vi "Create All Message Queues Sample Panel.vi"(8 "error in (no error)":cluster{"状态":bool, "代码":i32, "源":string} caption="错误输入（无错误）") -> (0 "error out":cluster{"状态":bool, "代码":i32, "源":string} caption="错误输出", 3 "消息队列":T1)   [LabVIEW 2015, in "Message Queue.lvlib"]
doc: "本VI用于创建应用程序所需的所有消息队列。如应用程序需要两个以上消息队列，可右键单击上面的“消息队列”常量并选择打开自定义类型，将新的消息队列添加至该自定义类型，然后通过本VI进行初始化。"
uses:
  Message Queue.lvlib
  All Message Queues Sample Panel.ctl
  Message Cluster.ctl
  Enqueue Message (Single).vi
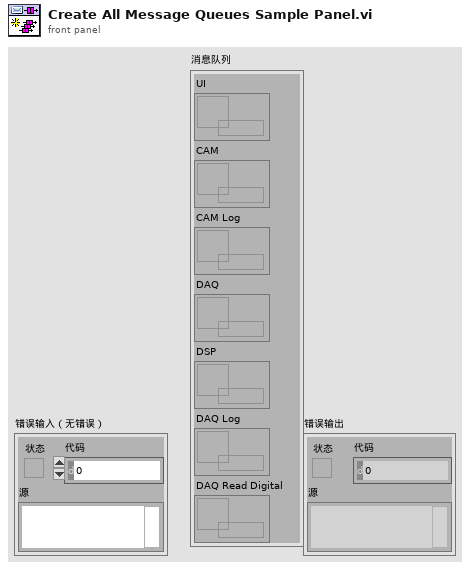
[diagram p1: front panel]
types:
  T1 = typedef "Message Queue.lvlib/All Message Queues Sample Panel.ctl" = cluster{"UI":refnum<queue>, "CAM":refnum<queue>, "CAM Log":refnum<queue>, "DAQ":refnum<queue>, "DSP":refnum<queue>, "DAQ Log":refnum<queue>, "DAQ Read Digital":refnum<queue>}
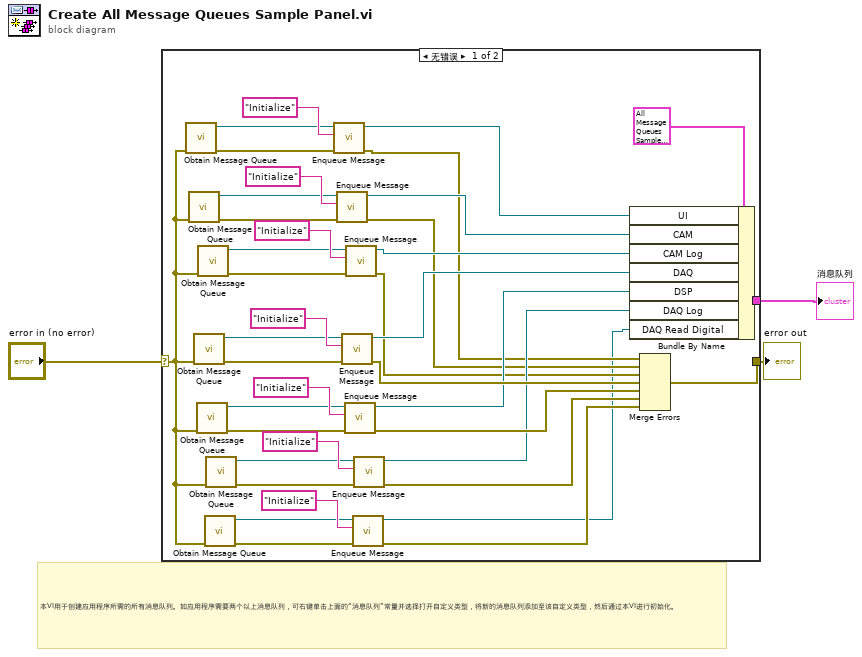
[diagram p0: block diagram]
diagram:
  # "本VI用于创建应用程序所需的所有消息队列。如应用程序需要两个以上消息队列，可右键单击上面的“消息队列”常量并选择打开自定义类型，将新的消息队列添加至该自定义类型，然后通过本VI进行初始化。"
  n1 = case shown="无错误" "error in (no error)" {
    selector: "error in (no error)" -> [w6 w43]
    tunnel: [w35 w43] -> w3
    tunnel: [w42 _] -> w1
    frame No Error {
      n2 = call "Obtain Message Queue.vi"("error in (no error)"=w6) -> ("error out"=w24:cluster{"状态":bool, "代码":i32, "源":string}, "消息队列"=w22:refnum<queue>)  [unwired: 9 in]
      n3 = call "Obtain Message Queue.vi"("error in (no error)"=w6) -> ("error out"=w21:cluster{"状态":bool, "代码":i32, "源":string}, "消息队列"=w19:refnum<queue>)  [unwired: 9 in]
      n4 = call "Obtain Message Queue.vi"("error in (no error)"=w6) -> ("error out"=w41:cluster{"状态":bool, "代码":i32, "源":string}, "消息队列"=w39:refnum<queue>)  [unwired: 9 in]
      n5 = call "Obtain Message Queue.vi"("error in (no error)"=w6) -> ("error out"=w38:cluster{"状态":bool, "代码":i32, "源":string}, "消息队列"=w36:refnum<queue>)  [unwired: 9 in]
      n6 = call "Obtain Message Queue.vi"("error in (no error)"=w6) -> ("error out"=w18:cluster{"状态":bool, "代码":i32, "源":string}, "消息队列"=w16:refnum<queue>)  [unwired: 9 in]
      n7 = call "Obtain Message Queue.vi"("error in (no error)"=w6) -> ("error out"=w9:cluster{"状态":bool, "代码":i32, "源":string}, "消息队列"=w7:refnum<queue>)  [unwired: 9 in]
      n8 = call "Obtain Message Queue.vi"("error in (no error)"=w6) -> ("error out"=w30:cluster{"状态":bool, "代码":i32, "源":string}, "消息队列"=w28:refnum<queue>)  [unwired: 9 in]
      n9 = call-poly "Enqueue Message.vi"("error in (no error)"=w24, "消息"="Initialize" ("Message"), "消息队列"=w22) -> ("error out"=w12:cluster{"状态":bool, "代码":i32, "源":string}, "消息队列副本"=w13:refnum<queue>)  [unwired: 7 in]
      n10 = call-poly "Enqueue Message.vi"("error in (no error)"=w21, "消息"="Initialize" ("Message"), "消息队列"=w19) -> ("error out"=w11:cluster{"状态":bool, "代码":i32, "源":string}, "消息队列副本"=w14:refnum<queue>)  [unwired: 7 in]
      n11 = call-poly "Enqueue Message.vi"("error in (no error)"=w41, "消息"="Initialize" ("Message"), "消息队列"=w39) -> ("error out"=w34:cluster{"状态":bool, "代码":i32, "源":string}, "消息队列副本"=w31:refnum<queue>)  [unwired: 7 in]
      n12 = call-poly "Enqueue Message.vi"("error in (no error)"=w38, "消息"="Initialize" ("Message"), "消息队列"=w36) -> ("error out"=w33:cluster{"状态":bool, "代码":i32, "源":string}, "消息队列副本"=w32:refnum<queue>)  [unwired: 7 in]
      n13 = call-poly "Enqueue Message.vi"("error in (no error)"=w18, "消息"="Initialize" ("Message"), "消息队列"=w16) -> ("error out"=w10:cluster{"状态":bool, "代码":i32, "源":string}, "消息队列副本"=w15:refnum<queue>)  [unwired: 7 in]
      n14 = call-poly "Enqueue Message.vi"("error in (no error)"=w9, "消息"="Initialize" ("Message"), "消息队列"=w7) -> ("error out"=w5:cluster{"状态":bool, "代码":i32, "源":string}, "消息队列副本"=w4:refnum<queue>)  [unwired: 7 in]
      n15 = call-poly "Enqueue Message.vi"("error in (no error)"=w30, "消息"="Initialize" ("Message"), "消息队列"=w28) -> ("error out"=w26:cluster{"状态":bool, "代码":i32, "源":string}, "消息队列副本"=w27:refnum<queue>)  [unwired: 7 in]
      n16 = Bundle By Name(cluster=T1 {"UI"=refnum, "CAM"=refnum, "CAM Log"=refnum, "DAQ"=refnum, "DSP"=refnum, "DAQ Log"=refnum, "DAQ Read Digital"=refnum} ("消息队列"), "UI"=w13, "CAM"=w14, "CAM Log"=w15, "DAQ"=w31, "DSP"=w32, "DAQ Log"=w27, "DAQ Read Digital"=w4) -> (w42:T1)
      n17 = Merge Errors(w12, w11, w10, w34, w33, w26, w5) -> (w35:errorcluster)
    }
    frame Error {
    }
  }
  "error out" <- w3
  "消息队列" <- w1
